vi "TreeMenuUpdatePath.vi"(3 "error in":errorcluster, 4 "Level":i32, 5 "ProcessDataTreeMenu":refnum<vi>, 6 "stripped path":path) -> (0 "error out":errorcluster, 2 "stripped path out":path)   [LabVIEW 2013, in "main.lvlib"]
uses:
  main.lvlib
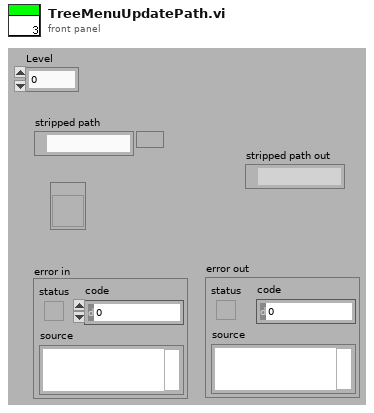
[diagram p1: front panel]
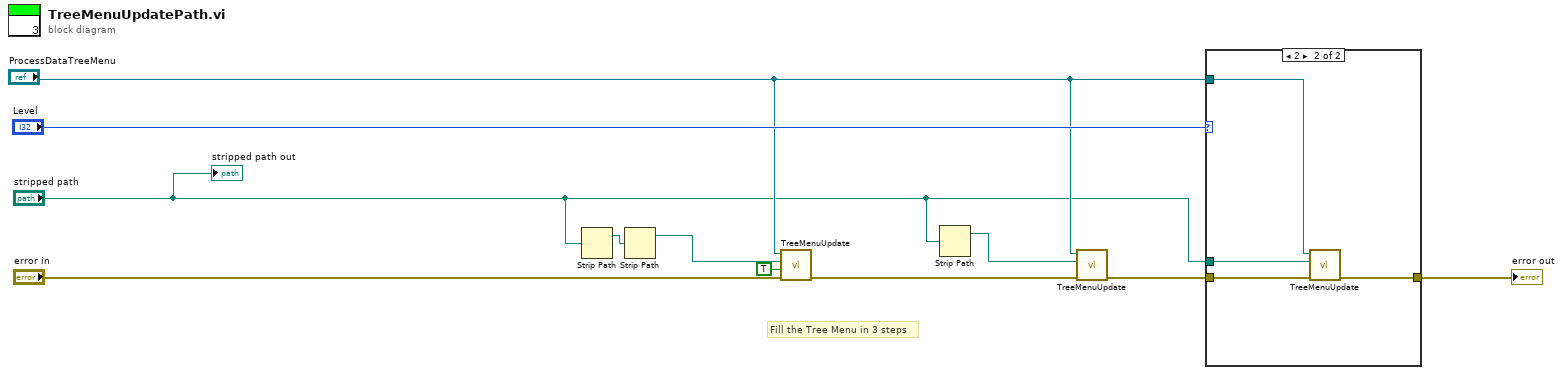
[diagram p0: block diagram]
diagram:
  # "Fill the Tree Menu in 3 steps"
  n1 = Strip Path(path="stripped path") -> (stripped path=w7:path)  [unwired: 1 out]
  n2 = Strip Path(path=w7) -> (stripped path=w6:path)  [unwired: 1 out]
  n3 = call "TreeMenuUpdate.vi"("error in"="error in", "Date?"=TRUE ("CPR?"), "stripped path"=w6, "Tree Refnum"="ProcessDataTreeMenu") -> ("error out"=w8:errorcluster)  [unwired: 3 in]
  n4 = Strip Path(path="stripped path") -> (stripped path=w11:path)  [unwired: 1 out]
  n5 = call "TreeMenuUpdate.vi"("error in"=w8, "stripped path"=w11, "Tree Refnum"="ProcessDataTreeMenu") -> ("error out"=w10:errorcluster)  [unwired: 4 in]
  n6 = case shown="2" "Level" {
    tunnel: w10 -> [w12 w16]
    tunnel: [w12 w15] -> w9
    tunnel: "ProcessDataTreeMenu" -> [_ w14]
    tunnel: "stripped path" -> [_ w13]
    frame 0, Default {
    }
    frame 2 {
      n7 = call "TreeMenuUpdate.vi"("error in"=w16, "stripped path"=w13, "Tree Refnum"=w14) -> ("error out"=w15:errorcluster)  [unwired: 4 in]
    }
  }
  "error out" <- w9
  "stripped path out" <- "stripped path"
